vi "Fundamental Vector (N Channels).vi"(8 "error in (no error)":errorcluster, 10 "current waveforms":waveform(dbl)[](array[waveform]), 11 "voltage waveforms":waveform(dbl)[](array[waveform])) -> (0 "error out":errorcluster, 2 "current fundamental vectors":cdb[](array[numeric]), 3 "voltage fundamental vectors":cdb[](array[numeric]), 5 "frequency":dbl)   [LabVIEW 2014, in "NI_EP_Basic.lvlib"]
doc: "Calculates the fundamental vector of a voltage or current signal. Wire data to the <B>voltage waveform</B> input or the <B>current waveform</B> input to determine the polymorphic instance to use or manually select the instance."
uses:
  <vilib>/addons/Electrical Power/Basic/NI_EP_Basic.lvlib
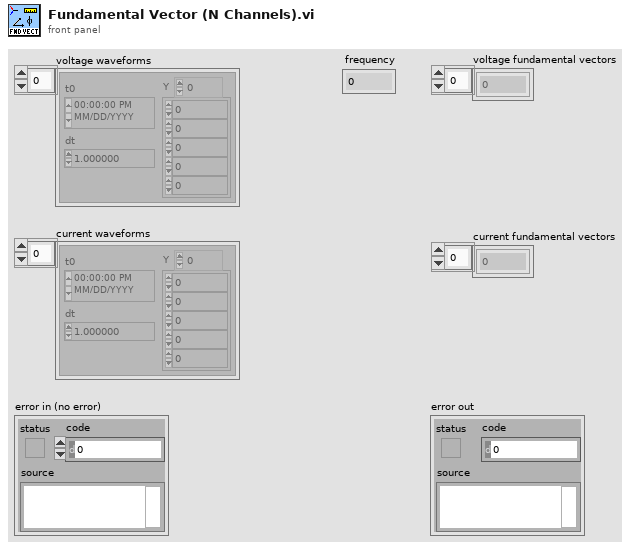
[diagram p1: front panel]
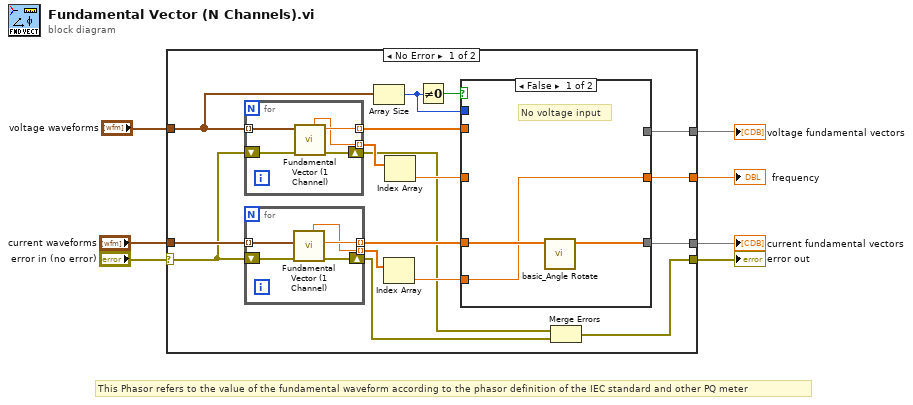
[diagram p0: block diagram]
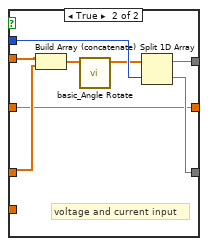
[diagram p2: hidden frame]
diagram:
  # "This Phasor refers to the value of the fundamental waveform according to the phasor definition of the IEC standard and other PQ meter"
  n1 = case shown="No Error" "error in (no error)" {
    selector: "error in (no error)" -> [w23 w46]
    tunnel: "voltage waveforms" -> [w8 _]
    tunnel: "current waveforms" -> [w24 _]
    tunnel: [w18 _] -> w4
    tunnel: [w14 _] -> w3
    tunnel: [w11 w46] -> w2
    tunnel: [w10 _] -> w1
    frame No Error {
      n2 = for {
        tunnel: w8 -> [w45] mode=indexing
        shift-right: [w42] -> w13
        shift-left: w23 -> [w44]
        tunnel: [w43] -> w17 mode=indexing
        tunnel: [w41] -> w21 mode=indexing
        n3 = call <vilib>:"Fundamental Vector (1 Channel).vi"("error in (no error)"=w44, "voltage waveform"=w45) -> ("error out"=w42:errorcluster, "voltage fundamental vector"=w43:cdb, "frequency"=w41:dbl)  [unwired: 6 in, 1 out]
      }
      n4 = for {
        tunnel: w24 -> [w40] mode=indexing
        shift-right: [w37] -> w12
        shift-left: w23 -> [w39]
        tunnel: [w38] -> w16 mode=indexing
        tunnel: [w36] -> w22 mode=indexing
        n5 = call <vilib>:"Fundamental Vector (1 Channel).vi"("error in (no error)"=w39, "current waveform"=w40) -> ("error out"=w37:errorcluster, "current fundamental vector"=w38:cdb, "frequency"=w36:dbl)  [unwired: 6 in, 1 out]
      }
      n6 = Array Size(array=w8) -> (size(s)=w9:i32)
      n7 = Index Array(array=w22) -> (element=w15:dbl)  [unwired: 1 in]
      n8 = Index Array(array=w21) -> (element=w19:dbl)  [unwired: 1 in]
      n9 = Not Equal To 0?(x=w9) -> (x != 0?=w20:bool)
      n10 = case shown="False" w20 {
        tunnel: w19 -> [_ w28]
        tunnel: [w25 w28] -> w18
        tunnel: w17 -> [_ w35]
        tunnel: [w26 w31] -> w14
        tunnel: w16 -> [w27 w34]
        tunnel: w15 -> [w25 _]
        tunnel: [_ w33] -> w10
        tunnel: w9 -> [_ w32]
        frame False {
          # "No voltage input"
          n11 = call <vilib>:"basic_Angle Rotate.vi"("array in"=w27) -> ("array out"=w26:cdb[])  [unwired: 10 in]
        }
        frame True {
          # "voltage and current input"
          n12 = Build Array (concatenate)(w35, w34) -> (w30:cdb[])
          n13 = call <vilib>:"basic_Angle Rotate.vi"("array in"=w30) -> ("array out"=w29:cdb[])  [unwired: 10 in]
          n14 = Split 1D Array(array=w29, index=w32) -> (first subarray=w33:cdb[], second subarray=w31:cdb[])
        }
      }
      n15 = Merge Errors(w13, w12) -> (w11:errorcluster)
    }
    frame Error {
    }
  }
  "voltage fundamental vectors" <- w1
  "frequency" <- w4
  "error out" <- w2
  "current fundamental vectors" <- w3
